vi "ColormapToIntensityGraphZMarkers.vi"(0 "Colormap":T1=enum."None ", 1 "Input Colormap":T2={"Max"=16777215, "Min"=0, "Median"=8816262, "Overflow"=0, "Underflow"=0, "Interpolate"=TRUE, "Show Underflow"=FALSE, "Show Overflow"=FALSE, "Undeflow\n(% of med)"=0.0, "Overlow \n(% of med)"=0.0}, 5 "Min":dbl, 7 "Median":dbl=5.0, 9 "Max":dbl=255.0) -> (4 "Z Scale.Marker Values[]":cluster{dbl, u32}[](array[cluster])=[{0.0, 0}, {5.0, 0}, {255.0, 0}])   [LabVIEW 2017]
uses:
  ColorMapDataType.ctl
  ColorMapEnum.ctl
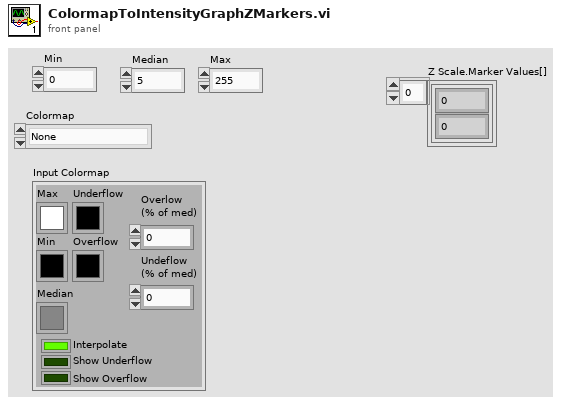
[diagram p1: front panel]
types:
  T1 = typedef "ColorMapEnum.ctl" = enum16{"high_low grayscale", "grayscale", "jet", "high_low_winter", "None "}
  T2 = typedef "ColorMapDataType.ctl" = cluster{"Max":u32, "Min":u32, "Median":u32, "Overflow":u32, "Underflow":u32, "Interpolate":bool, "Show Underflow":bool, "Show Overflow":bool, "Undeflow\n(% of med)":dbl, "Overlow \n(% of med)":dbl}
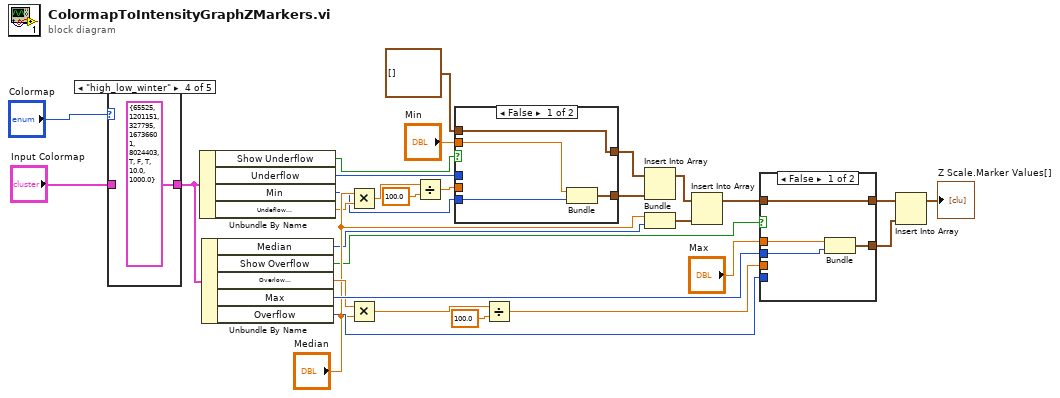
[diagram p0: block diagram]
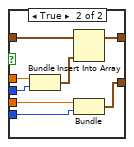
[diagram p2: hidden frame]
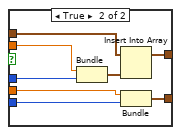
[diagram p3: hidden frame]
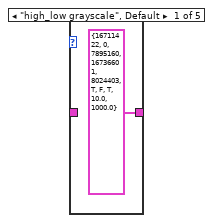
[diagram p4: hidden frame]
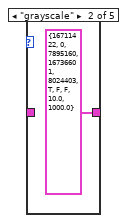
[diagram p5: hidden frame]
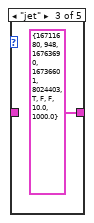
[diagram p6: hidden frame]
diagram:
  n1 = case shown="\"high_low_winter\"" "Colormap" {
    tunnel: [T2 {"Max"=16711422, "Min"=0, "Median"=7895160, "Overflow"=16736601, "Underflow"=8024403, "Interpolate"=TRUE, "Show Underflow"=FALSE, "Show Overflow"=TRUE, "Undeflow\n(% of med)"=10.0, "Overlow \n(% of med)"=1000.0} ("Colormap") T2 {"Max"=16711422, "Min"=0, "Median"=7895160, "Overflow"=16736601, "Underflow"=8024403, "Interpolate"=TRUE, "Show Underflow"=FALSE, "Show Overflow"=FALSE, "Undeflow\n(% of med)"=10.0, "Overlow \n(% of med)"=1000.0} ("Colormap") T2 {"Max"=16711680, "Min"=948, "Median"=16763690, "Overflow"=16736601, "Underflow"=8024403, "Interpolate"=TRUE, "Show Underflow"=FALSE, "Show Overflow"=FALSE, "Undeflow\n(% of med)"=10.0, "Overlow \n(% of med)"=1000.0} ("Colormap") T2 {"Max"=65525, "Min"=1201151, "Median"=327795, "Overflow"=16736601, "Underflow"=8024403, "Interpolate"=TRUE, "Show Underflow"=FALSE, "Show Overflow"=TRUE, "Undeflow\n(% of med)"=10.0, "Overlow \n(% of med)"=1000.0} ("Colormap") w35] -> w14
    tunnel: "Input Colormap" -> [_ _ _ _ w35]
    frame "high_low grayscale", Default {
    }
    frame "grayscale" {
    }
    frame "jet" {
    }
    frame "high_low_winter" {
    }
    frame "None " {
    }
  }
  n2 = Unbundle By Name(w14) -> ("Show Underflow"=w2:bool, "Underflow"=w6:u32, "Min"=w8:u32, "Undeflow\n(% of med)"=w11:dbl)
  n3 = Unbundle By Name(w14) -> ("Median"=w15:u32, "Show Overflow"=w18:bool, "Overlow \n(% of med)"=w22:dbl, "Max"=w25:u32, "Overflow"=w26:u32)
  n4 = Multiply(x="Median", y=w11) -> (x*y=w9:dbl)
  n5 = Multiply(x=w22, y="Median") -> (x*y=w19:dbl)
  n6 = Divide(x=w9, y=100.0) -> (x/y=w12:dbl)
  n7 = case shown="False" w2 {
    tunnel: cluster{dbl, u32}[] [] ("Z Scale.Marker Values[]") -> [w39 w47]
    tunnel: [w39 w46] -> w7
    tunnel: "Min" -> [w37 w45]
    tunnel: w6 -> [_ w44]
    tunnel: w8 -> [w38 w42]
    tunnel: w12 -> [_ w41]
    tunnel: [w36 w40] -> w13
    frame False {
      n8 = Bundle("Min"=w37, "Min"=w38) -> (w36:cluster{"Min":dbl, "Min":u32})  [unwired: 1 in]
    }
    frame True {
      n9 = Bundle("Min"=w45, "Underflow"=w44) -> (w43:cluster{"Min":dbl, "Underflow":u32})  [unwired: 1 in]
      n10 = Insert Into Array(array=w47, new element=w43) -> (w46:cluster{dbl, u32}[])  [unwired: 1 in]
      n11 = Bundle(w41, "Min"=w42) -> (w40:cluster{dbl, "Min":u32})  [unwired: 1 in]
    }
  }
  n12 = Divide(x=w19, y=100.0) -> (x/y=w23:dbl)
  n13 = Insert Into Array(array=w7, new element=w13) -> (w17:cluster{dbl, u32}[])  [unwired: 1 in]
  n14 = Bundle("Median"="Median", "Median"=w15) -> (w16:cluster{"Median":dbl, "Median":u32})  [unwired: 1 in]
  n15 = Insert Into Array(array=w17, new element=w16) -> (w27:cluster{dbl, u32}[])  [unwired: 1 in]
  n16 = case shown="False" w18 {
    tunnel: w23 -> [_ w58]
    tunnel: [w50 w59] -> w29
    tunnel: "Max" -> [w49 w57]
    tunnel: w25 -> [w48 w56]
    tunnel: w26 -> [_ w55]
    tunnel: w27 -> [w51 w54]
    tunnel: [w51 w52] -> w28
    frame False {
      n17 = Bundle("Max"=w49, "Max"=w48) -> (w50:cluster{"Max":dbl, "Max":u32})  [unwired: 1 in]
    }
    frame True {
      n18 = Bundle("Max"=w57, "Max"=w56) -> (w53:cluster{"Max":dbl, "Max":u32})  [unwired: 1 in]
      n19 = Insert Into Array(array=w54, new element=w53) -> (w52:cluster{dbl, u32}[])  [unwired: 1 in]
      n20 = Bundle(w58, "Overflow"=w55) -> (w59:cluster{dbl, "Overflow":u32})  [unwired: 1 in]
    }
  }
  n21 = Insert Into Array(array=w28, new element=w29) -> (→"Z Scale.Marker Values[]":cluster{dbl, u32}[])  [unwired: 1 in]
